vi "AG6000A Load Setup.vi"(8 "error in (no error)":errorcluster {"code" format="%.0x"}, 10 "Setup to Load":string(combo)="CH1", 11 "VISA session":refnum<visa-resource-name>) -> (0 "error out":errorcluster {"code" format="%.0x"}, 3 "dup VISA session":refnum<visa-resource-name>)   [LabVIEW 2020]
doc: "This VI configures the oscilloscope to perform a continuous acquisition."
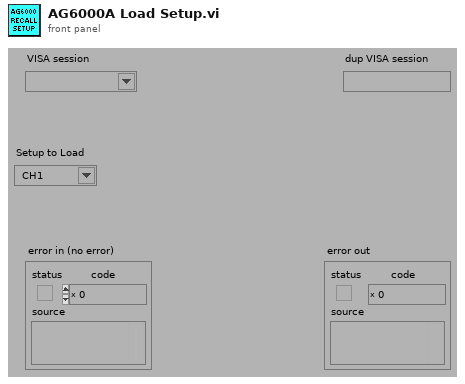
[diagram p1: front panel]
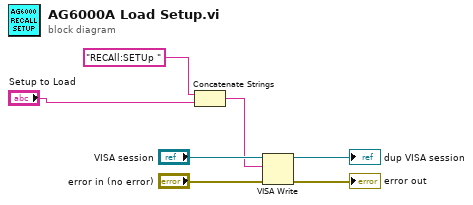
[diagram p0: block diagram]
diagram:
  n1 = Concatenate Strings("RECAll:SETUp " ("string (\"\")"), "Setup to Load") -> (w2:string)
  n2 = VISA Write(VISA resource name="VISA session", write buffer=w2, error in (no error)="error in (no error)") -> (VISA resource name out=→"dup VISA session":refnum<visa-resource-name>, error out=→"error out":errorcluster)  [unwired: 1 out]
